vi "getHighlightedRows.vi"(8 "error in (no error)":errorcluster, 11 "GridDisplayable in":refnum<class "TransactionList.lvclass">) -> (0 "error out":errorcluster, 2 "Highlighted Rows":i32[](array[numeric]), 3 "GridDisplayable out":refnum<class "TransactionList.lvclass">)   [LabVIEW 2020, in "TransactionList.lvclass"]
uses:
  TransactionList.lvclass
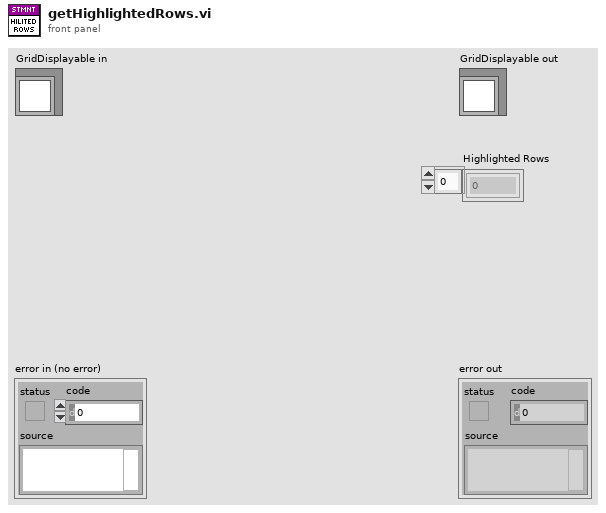
[diagram p1: front panel]
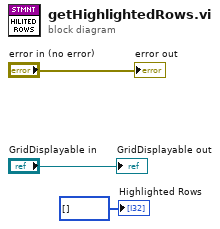
[diagram p0: block diagram]
diagram:
  "error out" <- "error in (no error)"
  "GridDisplayable out" <- "GridDisplayable in"
  "Highlighted Rows" <- i32[] [] ("Highlighted Rows")
